vi "Behavior Wires Busy.vi"(0 "Sequence In":T1, 1 "Semaphore Number":i8) -> (7 "Sequence Out":T1)   [LabVIEW 2015]
doc: "Use this VI, in conjunction with the Wires array cluster, to restrict access to the Wires clusters to one operation at a time. This prevents simultaneous accessm which can cause, so called, Race Conditions i.e. errors due to multiple simutaneous writes."
uses:
  <vilib>/NXT/Subs/LVHSConnector.ctl
  <vilib>/NXT/LegoClasses/BrickReference/BrickReference.lvclass
  <vilib>/NXT/Dual Mode Library/Waits/Wait_NXTFlag.vi
  <vilib>/NXT/Dual Mode Library/Advanced/NXTFlag_Clear.vi
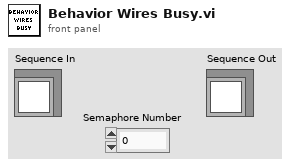
[diagram p1: front panel]
types:
  T1 = typedef "LVHSConnector.ctl" = refnum<class "BrickReference.lvclass">
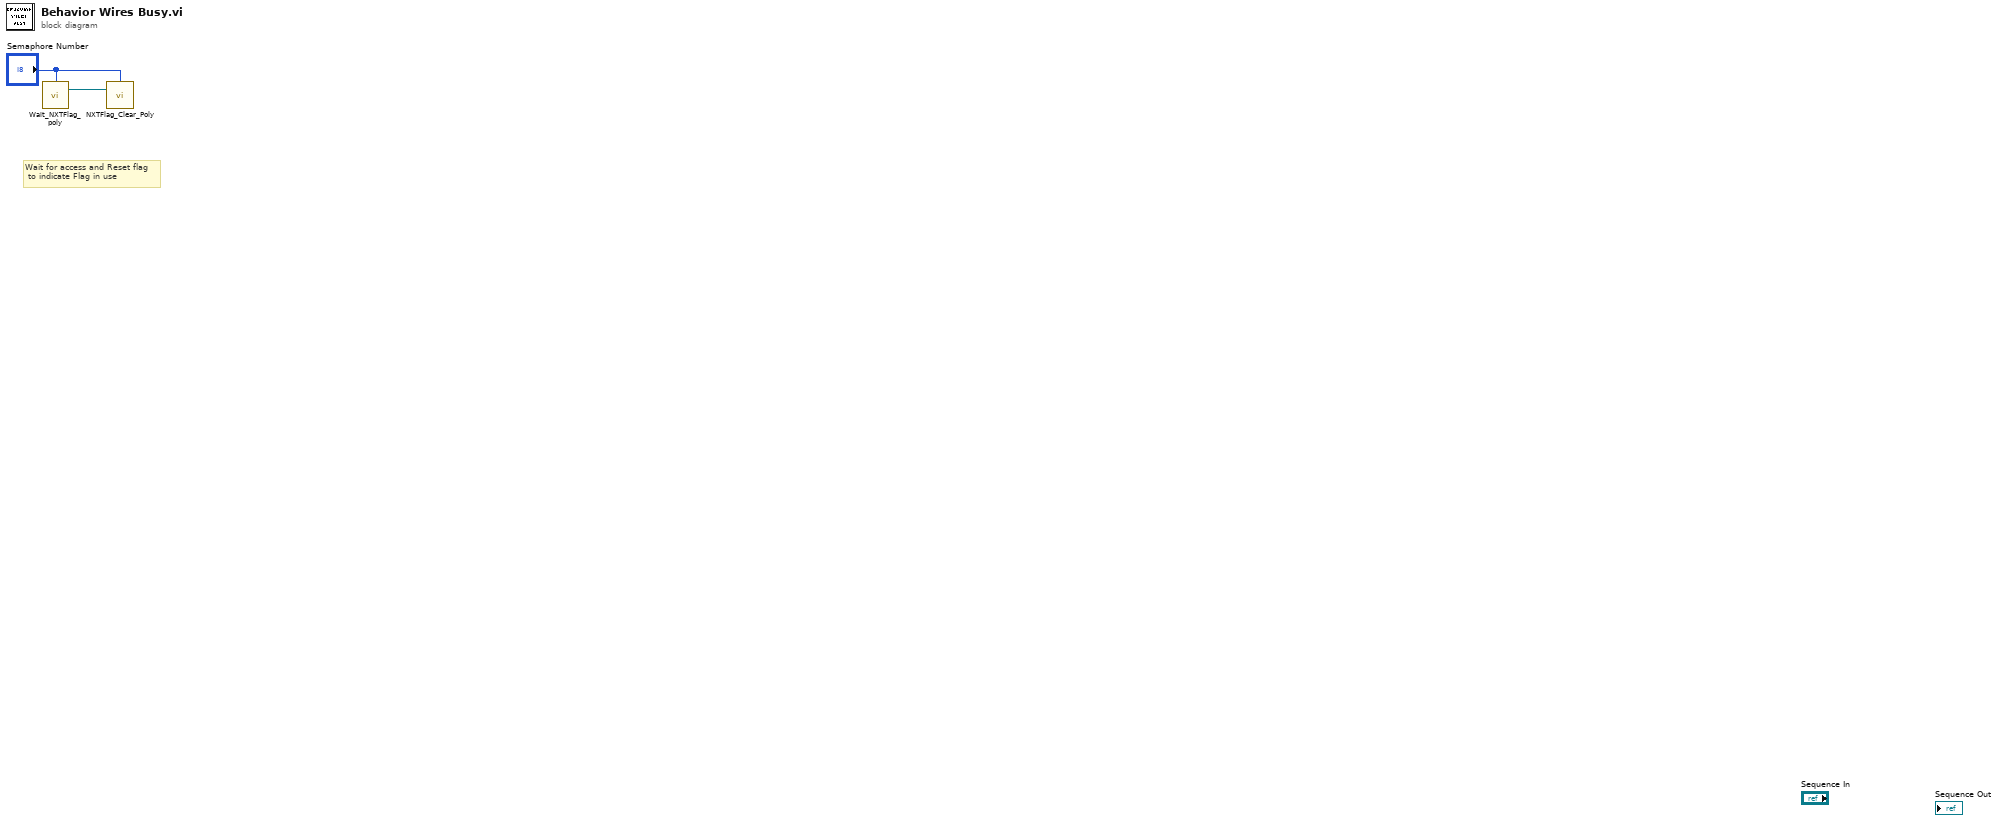
[diagram p0: block diagram]
diagram:
  # "Wait for access and Reset flag\n to indicate Flag in use"
  n1 = call-poly <vilib>:"Wait_NXTFlag_poly.vi"("NXT Flag Number"="Semaphore Number") -> ("NXT/EV3"=w1:T1)  [unwired: 3 in]
  n2 = call-poly <vilib>:"NXTFlag_Clear_Poly.vi"("NXT/EV3"=w1, "NXT/EV3 Flag Number"="Semaphore Number") -> ()  [unwired: 2 in, 1 out]
